vi "Parse Master Frame.vi"(8 "error in (no error)":errorcluster, 11 "Raw Master Line":string) -> (0 "error out":errorcluster, 1 "Record ID":u64, 2 "direction frame":string, 3 "speed frame":string, 10 "TIMESTAMP":u64)   [LabVIEW 2026]
uses:
  <vilib>/Utility/error.llb/Trim Whitespace (string).vi
  <vilib>/Utility/error.llb/Trim Whitespace One-Sided.vi
panel:
  out "Time Good?":bool
  out "HEX GOOD?":bool
  out "Length Good?":bool
  out "Record Good?":bool
  out "Type good?":bool
  out "Good?":bool
  out "Frame valid?":bool
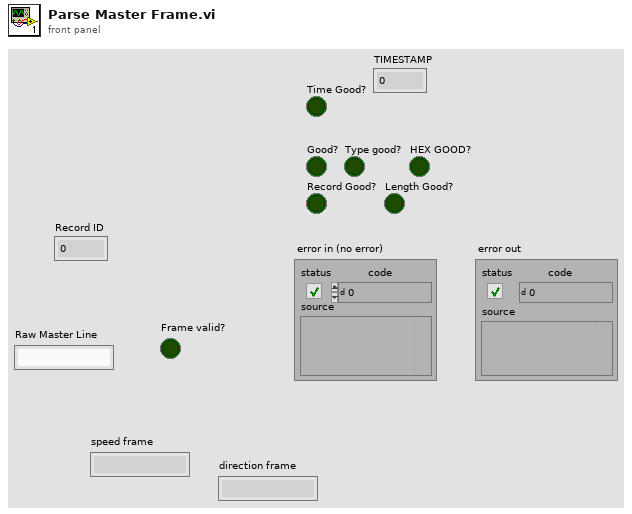
[diagram p1: front panel]
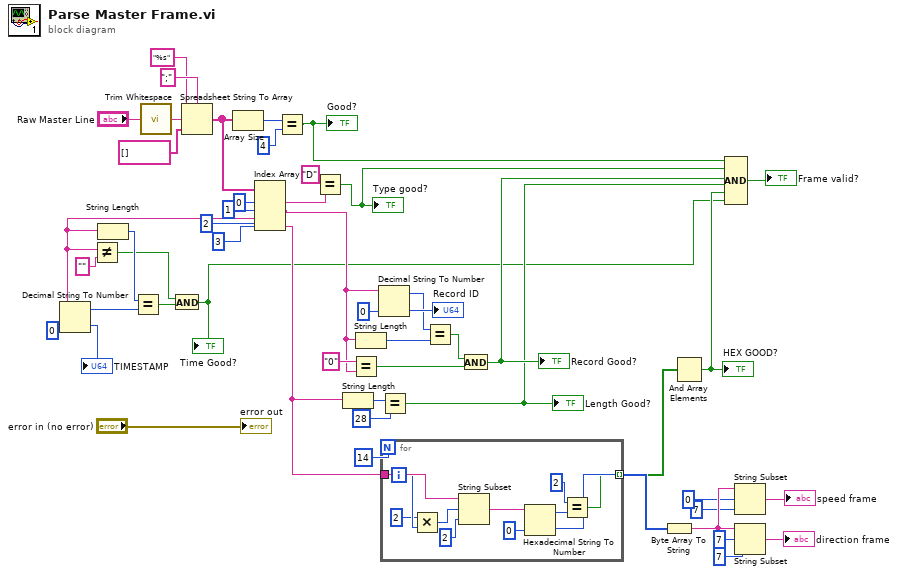
[diagram p0: block diagram]
diagram:
  n1 = call-poly <vilib>:"Trim Whitespace.vi"("string"="Raw Master Line") -> ("trimmed string"=w49:string)  [unwired: 1 in]
  n2 = Spreadsheet String To Array(delimiter (Tab)=";", format string="%s", spreadsheet string=w49, array type (2D Dbl)=string[] []) -> (array=w43:string[])
  n3 = Array Size(array=w43) -> (size(s)=w45:i32)
  n4 = Index Array(array=w43, index #1=0 ("index"), index #2=1 ("index"), index #3=2 ("index"), index #4=3 ("index")) -> (element #1=w41:string, element #2=w10:string, element #3=w2:string, element #4=w13:string)
  n5 = Decimal String To Number(string=w2, default (0L)=u64 0 ("default (0 I32)")) -> (offset past number=w8:i32, number=→"TIMESTAMP":u64)  [unwired: 1 in]
  n6 = Not Equal?(x=w2, y="") -> (x != y?=w4:bool)
  n7 = String Length(string=w2) -> (length=w6:i32)
  n8 = Equal?(x=w6, y=w8) -> (x = y?=w5:bool)
  n9 = And(x=w4, y=w5) -> (x .and. y?=w3:bool)
  "Time Good?" <- w3
  n10 = Equal?(x=w45, y=4) -> (x = y?=w22:bool)
  "Good?" <- w22
  n11 = Equal?(x=w41, y="D") -> (x = y?=w21:bool)
  "Type good?" <- w21
  n12 = String Length(string=w13) -> (length=w32:i32)
  n13 = Equal?(x="0", y=w10) -> (x = y?=w34:bool)
  n14 = String Length(string=w10) -> (length=w37:i32)
  n15 = Decimal String To Number(string=w10, default (0L)=u64 0 ("default (0 I32)")) -> (offset past number=w36:i32, number=→"Record ID":u64)  [unwired: 1 in]
  n16 = Equal?(x=w32, y=28) -> (x = y?=w19:bool)
  "Length Good?" <- w19
  n17 = for {
    N: 14 -> [_]
    tunnel: w13 -> [w62]
    tunnel: [w57] -> w29 mode=indexing
    tunnel: [w52] -> w28 mode=indexing
    i -> [w56]
    n18 = Multiply(x=2 ("y"), y=w56) -> (x*y=w61:i32)
    n19 = String Subset(string=w62, offset (0)=w61, length (rest)=2 ("length (rest)")) -> (substring=w59:string)
    n20 = Hexadecimal String To Number(string=w59, default (0uL)=u8 0 ("default (0 U32)")) -> (offset past number=w54:i32, number=w57:u8)  [unwired: 1 in]
    n21 = Equal?(x=2, y=w54) -> (x = y?=w52:bool)
  }
  n22 = Equal?(x=w36, y=w37) -> (x = y?=w33:bool)
  n23 = And(x=w33, y=w34) -> (x .and. y?=w20:bool)
  "Record Good?" <- w20
  n24 = Byte Array To String(unsigned byte array=w29) -> (string=w27:string)
  n25 = And Array Elements(Boolean array=w28) -> (logical AND=w18:bool)
  "HEX GOOD?" <- w18
  n26 = Compound Arithmetic op=AND(w22, w21, w20, w19, w18, w3) -> (→"Frame valid?":bool)
  n27 = String Subset(string=w27, offset (0)=0, length (rest)=7 ("length (rest)")) -> (substring=→"speed frame":string)
  n28 = String Subset(string=w27, offset (0)=7, length (rest)=7 ("length (rest)")) -> (substring=→"direction frame":string)
  "error out" <- "error in (no error)"
